vi "运维调试_CODMn.vi"() -> ()   [LabVIEW 2016, in "斯坦道CODMn新电路板.lvlib"]
uses:
  <vilib>/Utility/miscctls.llb/LVPointTypeDef.ctl
  <vilib>/Waveform/WDTFileIO.llb/Read Waveform from File.vi
  <vilib>/ptbypt/NI_PtbyPt.lvlib
panel:
  in  "告警代码":u16
  in  "周期设置":bool
  out "消解压力kPa":sgl format="%#.2f"
  out "权限等级":string
  out "总步数":i32
  out "滑动杆":u8(slide) caption="测试进度" scale=0.0..100.0
  in  "参数查询":bool
  in  "仪器校准":bool
  out "仪器版本号":string
  in  "试剂余量设置":bool
  out "试剂余量显示":sgl[][](graph)
  in  "公式切换阈值滴定数(0~9999)":dbl
  out "X0":u16
  in  "平台反控标样校准":enum16{"标液1", "标液2", "标液3"}(ring)
  in  "平台反控校准量程":enum16{"低量程1", "低量程2", "高量程1", "高量程2"}(ring)
  out "试剂传感器":sgl format="%#.2f"
  in  "历史波形 2":bool
  in  "返回 3":bool
  out "时间-温度":u16[](array[numeric]) caption="数组"
  out "温度波形时间":timestamp
  out "ORP滴定曲线 2":u16[](graph)
  in  "历史波形":bool
  in  "返回 2":bool
  out "滴定数-ORP值":u16[](array[numeric]) caption="数组"
  out "波形时间":timestamp
  out "ORP滴定曲线":u16[](graph)
  in  "滴定曲线":bool
  out "终点滴定数":sgl format="%#.2f"
  out "单位:":T1(ring)
  out "运行状态":T2 {"数据时间:" format="%<%y/%m/%d %H:%M:%S>T"; "仪器时间:" format="%<%y/%m/%d %H:%M:%S>T"}
  out "模块版本号":string
  out "当前步骤剩余时间":sgl format="%#.2f"
  out "加热实时温度":sgl format="%#.2f"
  out "ORP值/光值":sgl format="%#.2f"
  in  "布尔":bool
  in  "流程固件":bool
  in  "公式单个写入":bool
  in  "流程路径":path=path "C:/Users/STD/Documents/斯坦道流程文件/流程.xml"
  out "字符串":string
  out "运行时间":sgl format="%#.2f"
  out "环境湿度":sgl format="%#.2g"
  out "环境温度":sgl format="%#.2g"
  in  "数组":string[](array[string])
  in  "量程切换阈值写入":bool
  in  "量程切换阈值读取":bool
  in  "参数下拉列表":enum16{"CODMn"}(ring)
  in  "量程下拉列表":enum16{"低量程1", "低量程2", "高量程1", "高量程2"}(ring)
  in  "测量模式下拉列表":T3(ring)=enum."水样测量"
  in  "公式":cluster{"X^2":dbl, "X":dbl, "b":dbl}
  in  "写公式":bool
  in  "读公式":bool
  in  "返回":bool
  in  "设置":bool
  out "集成报警信息":string
  in  "停止":bool
  in  "手动启动":bool
  in  "单步测试":bool
  out "当前滴定数":sgl format="%#.2f"
  out "K":sgl format="%#.2f"
  out "B":sgl format="%#.2f"
  out "A":sgl format="%#.2f"
  out "多列列表框":i32(listbox)
  # "."
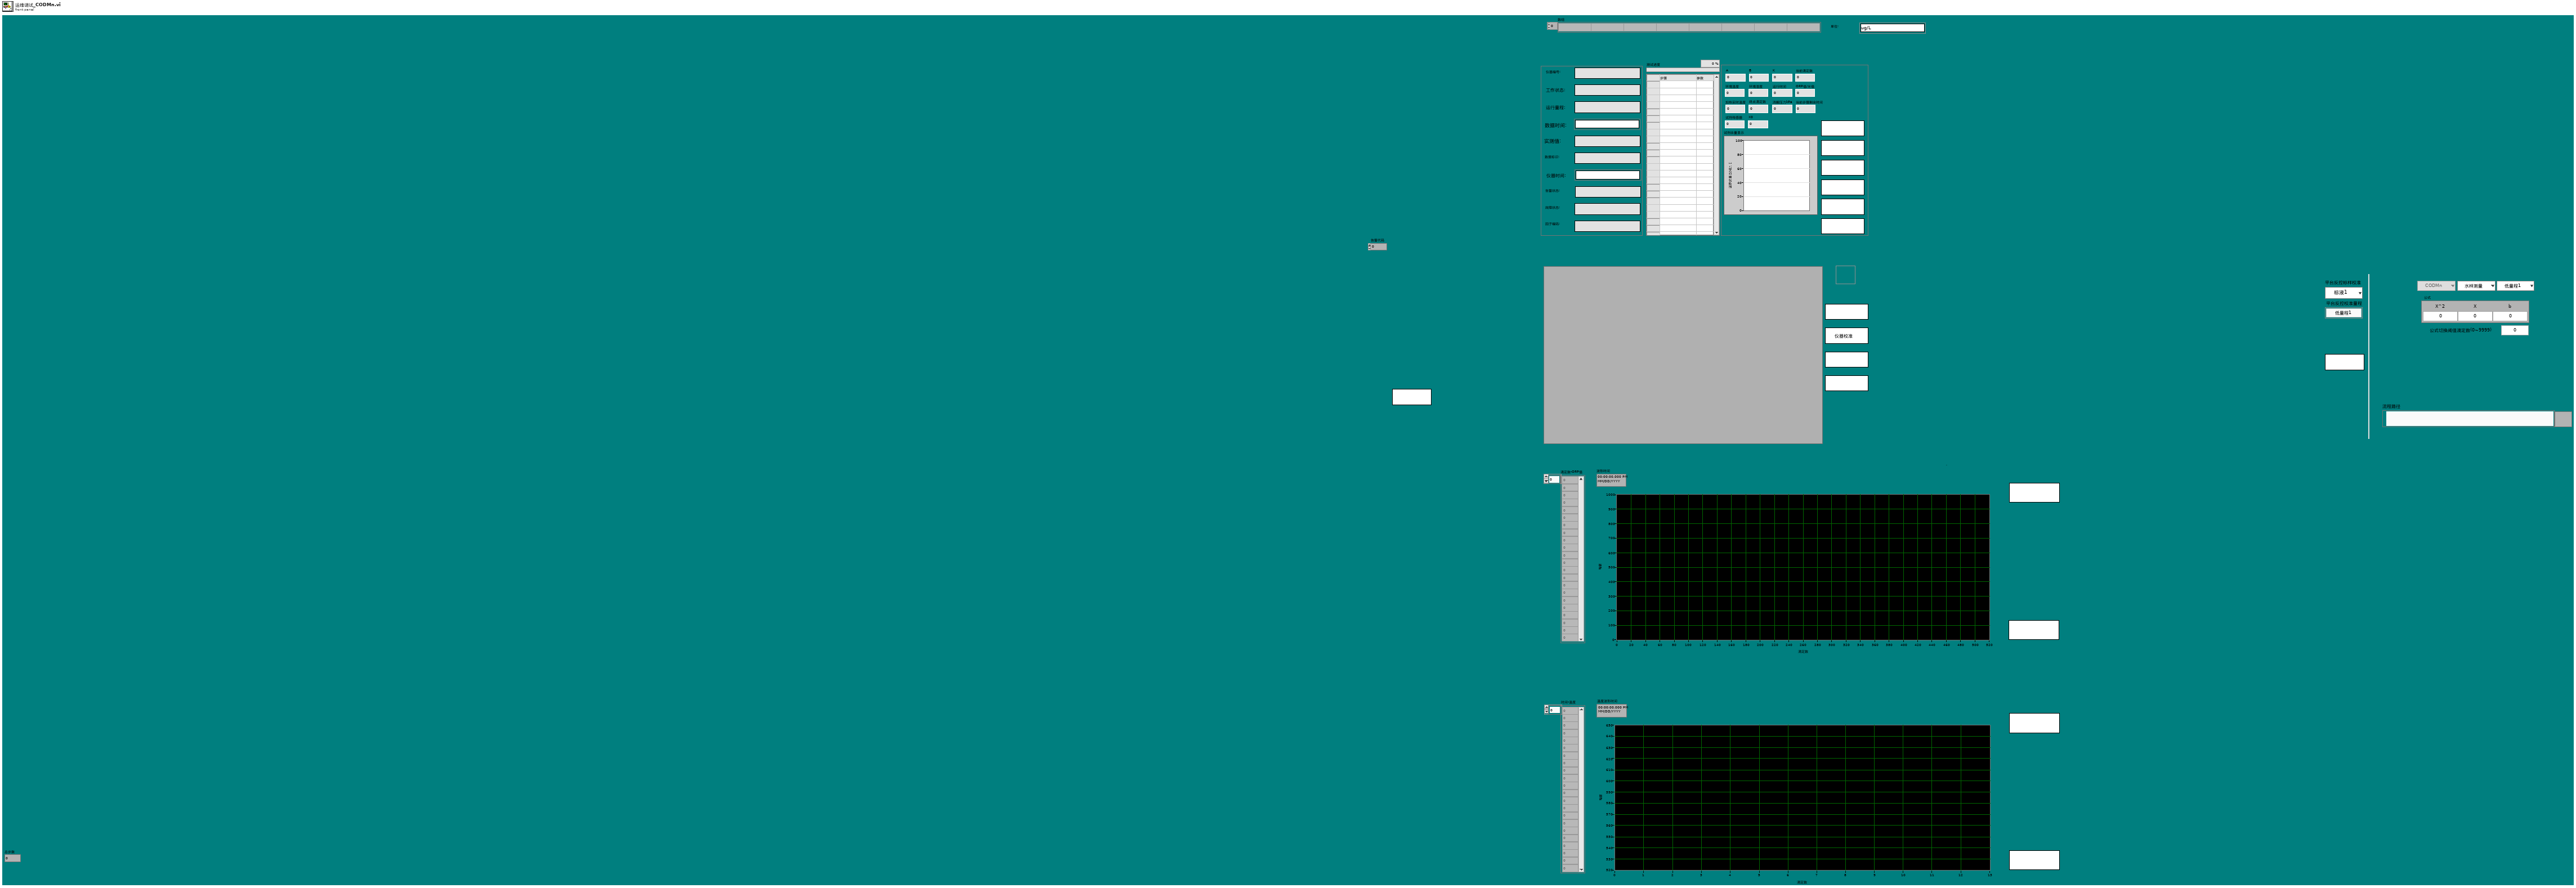
[diagram p1: front panel]
types:
  T1 = enum16{"ug/L", "mg/L", "ppm", "mg/m3", "cm", "ppb", "ug/m3", "%", "nmol/mol", "umol/mol", "MPN/L", "MPN/100ml", "ng/m3", "NTU", "无量纲", "ms/cm", "us/cm", "℃", "mV", "万个/L"}
  T2 = cluster{"仪器编号:":string, "工作状态:":string, "运行量程: ":string, "数据时间:":timestamp, "实测值:":string, "数据标识: ":string, "仪器时间:":timestamp, "告警状态: ":string, "故障状态:  ":string, "因子编码:":string}
  T3 = enum16{"", "水样测量", "标样核查", "零点核查", "跨度核查", "空白测试", "平行样测试", "加标回收"}
  T4 = cluster{"Major":u16, "Minor":u16, "Fix":u16, "Build":u16}
  T5 = cluster{"测量量程":sgl, "测量检出限":sgl, "测量精度":sgl, "测量间隔":sgl, "消解温度":sgl, "消解时长":sgl, "三项式系数":sgl, "二次多项式系数":sgl, "曲线斜率":sgl, "曲线截距":sgl, "线性相关系数":sgl, "空白校准时间":timestamp, "标样校准时间":timestamp, "测量信号值":sgl, "稀释倍数":sgl, "量程系数":sgl}
  T6 = typedef "LVPointTypeDef.ctl" = cluster{"Horizontal":i16, "Vertical":i16}
  T7 = cluster{"因子编码":u32, "单位":u16, "标样参考值":sgl, "水样数据时间":timestamp, "水样实测值":sgl, "水样数据标识":string, "标样数据时间":timestamp, "标样实测值":sgl, "标样数据标识":string, "空白数据时间":timestamp, "空白实测值":sgl, "空白数据标识":string, "零点核查数据时间":timestamp, "零点核查实测值":sgl, "零点核查数据标识":string, "跨度核查数据时间":timestamp, "跨度核查实测值":sgl, "跨度核查数据标识":string, "加标回收数据时间":timestamp, "加标回收实测值":sgl, "加标回收数据标识":string, "平行样数据时间":timestamp, "平行样实测值":sgl, "平行样数据标识":string, "F0":sgl, "F1":sgl, "F2":sgl, "F3":sgl, "F4":sgl, "F5":sgl, "F6":sgl, "F7":sgl, "温度":sgl, "湿度":sgl, "X值":sgl, "fidrange":u16}
  T8 = cluster{"系统时间":timestamp, "工作状态":u16, "测量模式":enum16{"待机", "连续模式", "周期模式", "定点模式", "受控模式", "手动模式"}, "告警代码":u16, "故障代码":u16, "日志代码":u16, "软件版本":u16, "A":sgl, "B":sgl, "K":sgl, "当前滴定数":sgl, "T":sgl, "H":sgl, "id":u16, "flowid":u16, "量程":u16, "加热实时温度":sgl, "当前ORP值":sgl, "运行时间":sgl, "当前步骤剩余时间":sgl, "结束滴定数":sgl, "注射泵保温温度":sgl, "匹配滴定数X0":u16, "X^2":sgl, "X":sgl, "B 2":sgl, "光值1":sgl, "光值2":sgl, "光值3":sgl, "光值4":sgl, "光值5":sgl, "光值6":sgl, "光值7":sgl, "光值8":sgl}
  T9 = cluster{"id":string, "ver":string, "type":string, "code":u16, "level":enum16{"一级", "二级", "三级"}, "message":string, "analysis":string, "platform_alarm_code":string}
  T10 = enum8{"Enabled", "Disabled", "Disabled and Grayed Out"}
  T11 = enum16{"空闲", "水样测试", "标样核查", "零点核查", "跨度核查", "空白测试", "平行样测试", "加标回收", "空白校准", "标样校准", "初始化（清洗）"}
  T12 = typedef "TimingControl.lvlib/TimingControl.lvclass/国标控制命令.ctl" = enum16{"启动测量", "标样核查", "零点核查", "跨度核查", "空白测试", "平行样测试", "加标回收", "空白校准", "标样校准", "初始化（清洗）", "停止测试", "仪器重启", "校时", "模式设置", "测量间隔设置"}
  T13 = typedef "TimingControl.lvlib/TimingControl.lvclass/测量参数.ctl" = u16
  T14 = cluster{"时间标识":timestamp, "设备":string, "日志信息":string, "流程参数":string}
  T15 = typedef "LVRowAndColumnUnsignedTypeDef.ctl" = cluster{"Row":u32, "Column":u32}
  T16 = enum32{"Bad", "Idle", "Run top level", "Running"}
  T17 = cluster{"站号":u16, "量程切换":enum32{"H", "L", "AUTO"}, "控制命令":u16, "模式设置":enum16{"待机", "连续模式", "周期模式", "定点模式", "受控模式", "手动模式"}, "测量间隔":u16}
  T18 = cluster{"测量量程":dbl, "测量精度":dbl, "测量间隔":dbl, "消解温度":dbl, "消解时长":dbl, "空白校准时间":timestamp, "曲线截距":dbl, "曲线斜率":dbl, "测量检出限":dbl, "测量信号值":dbl, "线性相关系数":dbl, "二次多项式系数":dbl, "标样校准时间":timestamp, "稀释倍数":dbl, "三项式系数":dbl, "空白标定系数":dbl, "量程系数":dbl, "F0/ORPA":dbl, "F1/ORPB":dbl, "F2/ORPK":dbl, "F3":dbl, "F4":dbl, "F5":dbl, "F6":dbl, "F7":dbl, "X0/滴定数":dbl, "量程":dbl}
  T19 = cluster{"跨度值":dbl, "零点标准液浓度":dbl, "跨度标准液浓度":dbl, "标准液标准浓度":dbl, "零点标准液偏差":dbl, "跨度标准液偏差":dbl, "标准液标准偏差":dbl}
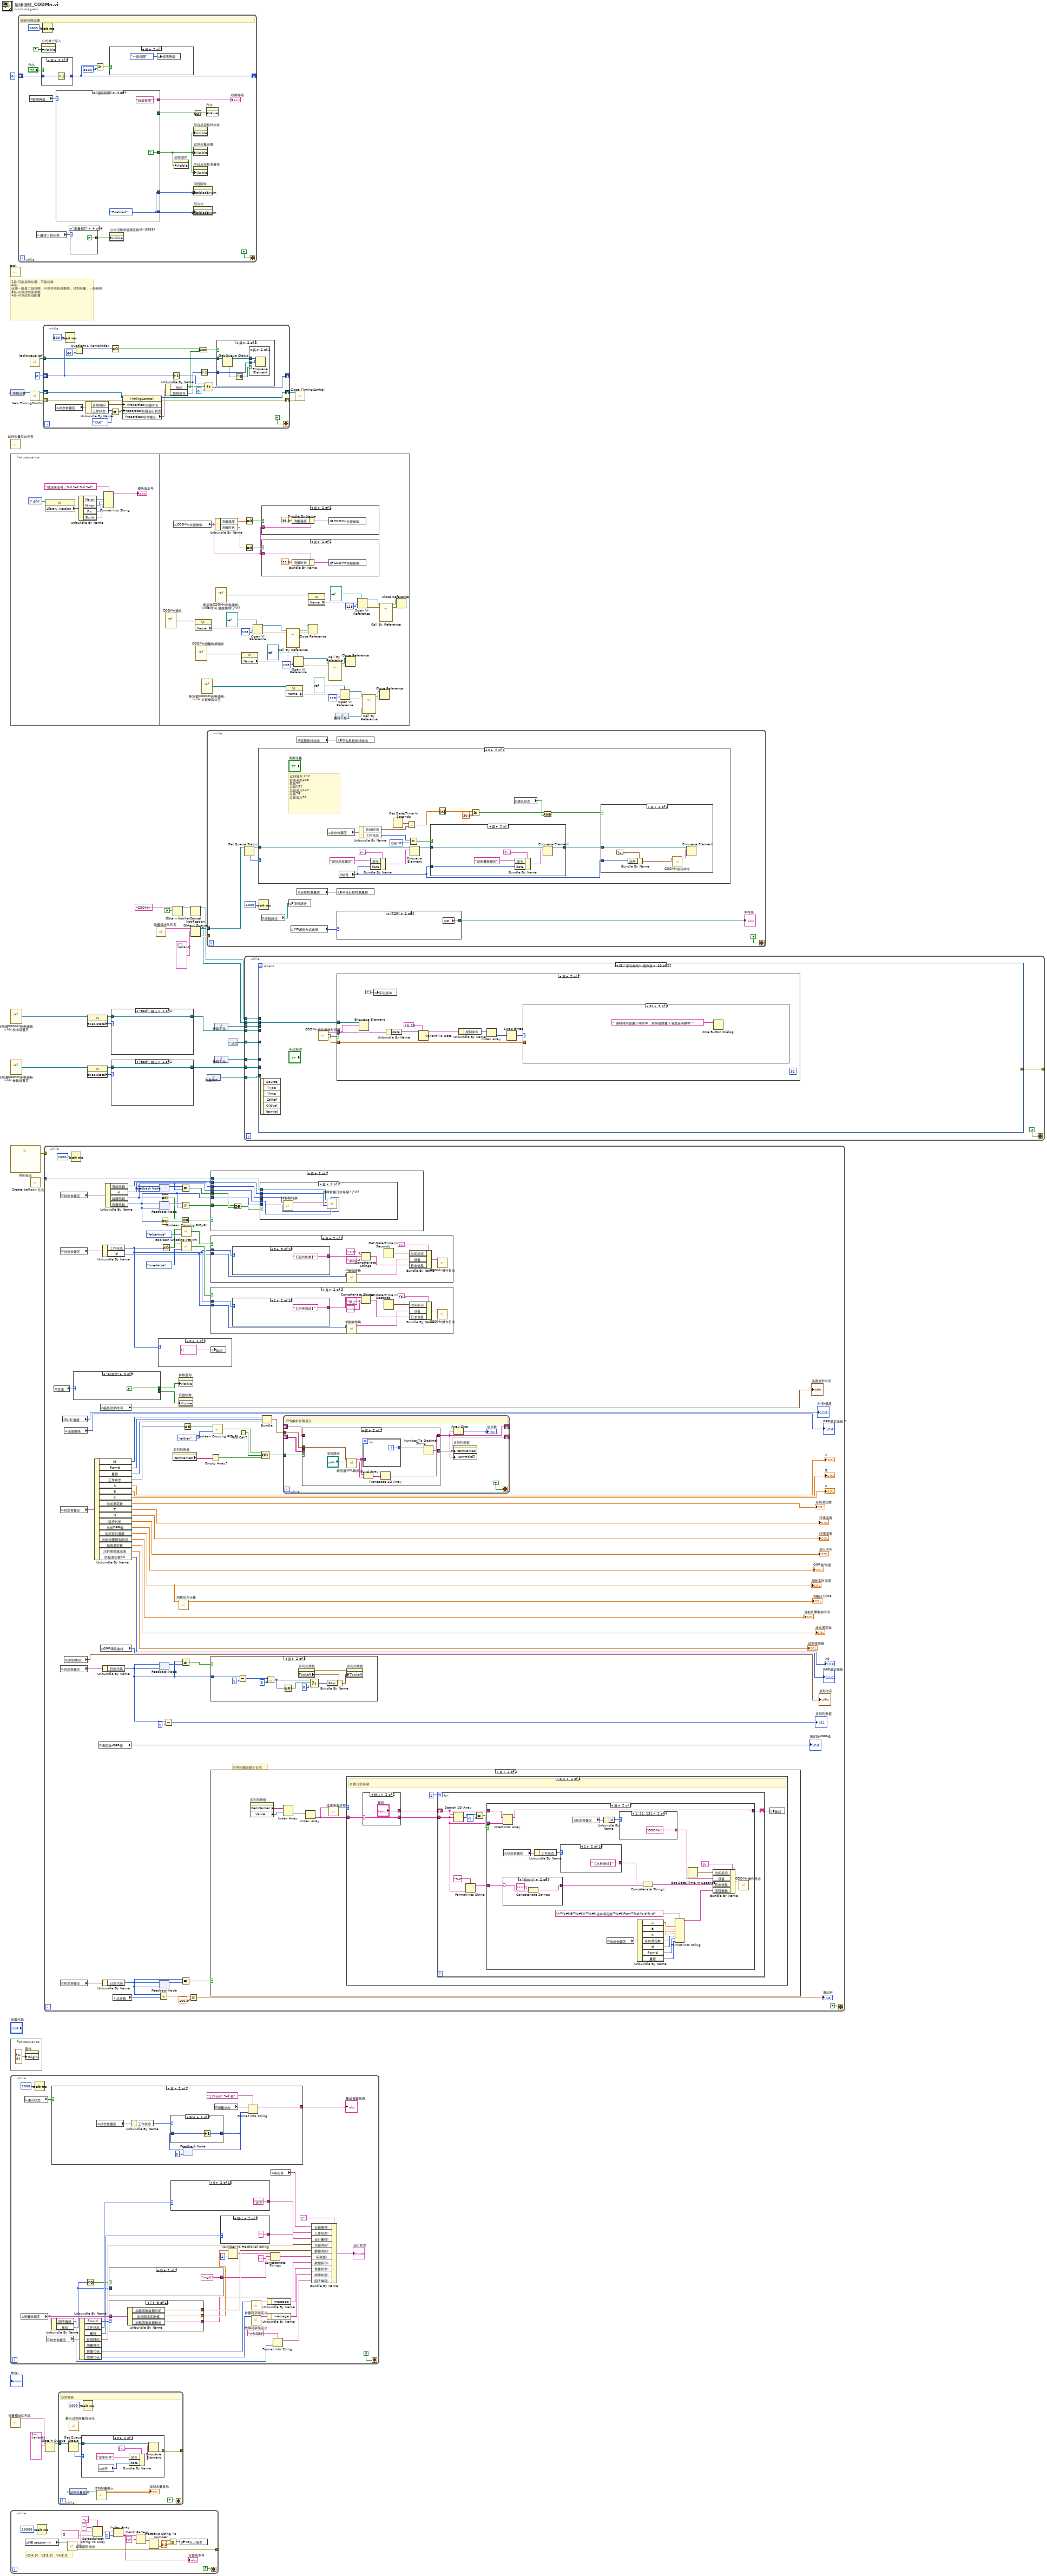
[diagram p0: block diagram]
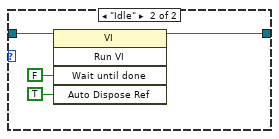
[diagram p2: hidden frame]
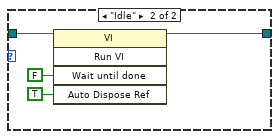
[diagram p3: hidden frame]
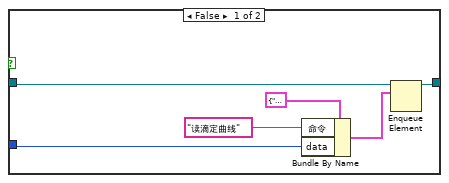
[diagram p6: hidden frame]
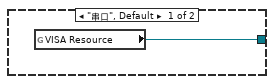
[diagram p8: hidden frame]
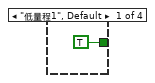
[diagram p11: hidden frame]
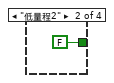
[diagram p12: hidden frame]
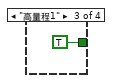
[diagram p13: hidden frame]
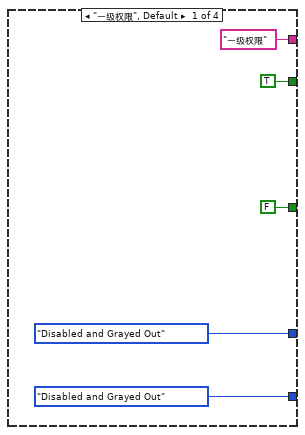
[diagram p14: hidden frame]
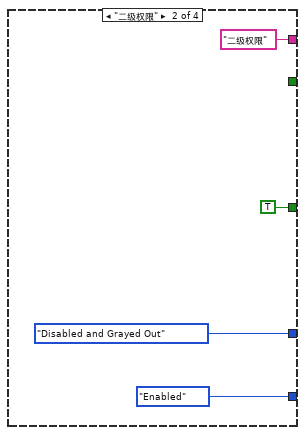
[diagram p15: hidden frame]
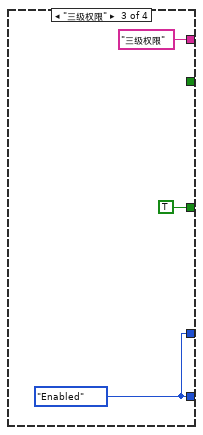
[diagram p16: hidden frame]
diagram:
  # "1级.只能启动仪器，不能校准\n2级.运维一般是二级权限，可以校准和改曲线，试剂余量，一般参数\n3级.可以改内部参数\n4级.可以改外设配置"
  n1 = call "task.vi"() -> ()  [unwired: 12 in]
  n2 = control-ref of="周期设置"() -> (w5:refnum<vi>)
  n3 = call "试剂余量后台任务.vi"() -> ()  [unwired: 12 in]
  n4 = flat-sequence {
    frame #0 {
      n5 = control-ref of="本VI"() -> (w41:refnum<vi>)
      n6 = property class="VI"(reference=w41) -> ("Library.Version"=w40:T4)  [unwired: 1 in, 2 out]
      n7 = Unbundle By Name(w40) -> ("Major"=w38:u16, "Minor"=w37:u16, "Fix"=w36:u16, "Build"=w35:u16)
      n8 = Format Into String(format string="模块版本号：%d.%d.%d.%d" ("格式字符串"), w38, w37, w36, w35) -> (resulting string=→"模块版本号":string)  [unwired: 2 in, 1 out]
    }
    frame #1 {
      n9 = vi-ref "CODMn通讯.vi"() -> (w55:refnum<vi>)
      n10 = global read "CODMn断电保存全局变量.vi" "CODMn关键参数"() -> (w42:T5)
      n11 = property class="VI"(reference=w55) -> ("Name"=w54:string)  [unwired: 1 in, 2 out]
      n12 = vi-ref "CODMn测量数据储存.vi"() -> (w79:refnum<vi>)
      n13 = vi-ref "斯坦道CODMn新电路板.lvlib:关键参数交互.vi"() -> (w65:refnum<vi>)
      n14 = Unbundle By Name(w42) -> ("消解温度"=w46:sgl, "消解时长"=w43:sgl)
      n15 = vi-ref "斯坦道CODMn新电路板.lvlib:时间-温度曲线(子VI).vi"() -> (w57:refnum<vi>)
      n16 = property class="VI"(reference=w79) -> ("Name"=w72:string)  [unwired: 1 in, 2 out]
      n17 = Equal To 0?(x=w46) -> (x = 0?=w45:bool)
      n18 = Equal To 0?(x=w43) -> (x = 0?=w44:bool)
      n19 = Open VI Reference(type specifier VI Refnum (for type only)=refnum<vi> refnum, vi path=w54, options=128 ("选项")) -> (vi reference=w52:refnum<vi>, error out=w50:errorcluster)  [unwired: 3 in]
      n20 = case shown="真" w45 {
        tunnel: w42 -> [_ w85]
        frame False {
        }
        frame True {
          n21 = Bundle By Name(cluster=w85, "消解温度"=sgl 95.0) -> (w84:T5)
          n22 = global write "CODMn断电保存全局变量.vi" "CODMn关键参数"(w84) -> ()
        }
      }
      n23 = case shown="真" w44 {
        tunnel: w42 -> [_ w82]
        frame False {
        }
        frame True {
          n24 = Bundle By Name(cluster=w82, "消解时长"=sgl 25.0) -> (w81:T5)
          n25 = global write "CODMn断电保存全局变量.vi" "CODMn关键参数"(w81) -> ()
        }
      }
      n26 = property class="VI"(reference=w65) -> ("Name"=w71:string)  [unwired: 1 in, 2 out]
      n27 = call-by-ref "?"(reference=w52, error in=w50) -> (reference out=w48:refnum<vi>, error out=w49:errorcluster)  [unwired: 12 in]
      n28 = Open VI Reference(type specifier VI Refnum (for type only)=refnum<vi> refnum, vi path=w72, options=128 ("选项")) -> (vi reference=w74:refnum<vi>, error out=w76:errorcluster)  [unwired: 3 in]
      n29 = property class="VI"(reference=w57) -> ("Name"=w63:string)  [unwired: 1 in, 2 out]
      n30 = Close Reference(reference=w48, error in (no error)=w49) -> ()  [unwired: 1 out]
      n31 = call-by-ref "?"(reference=w74, error in=w76) -> (reference out=w78:refnum<vi>, error out=w77:errorcluster)  [unwired: 12 in]
      n32 = control-ref of="量程下拉列表"() -> (w47:refnum<vi>)
      n33 = Open VI Reference(type specifier VI Refnum (for type only)=refnum<vi> refnum, vi path=w71, options=128 ("选项")) -> (vi reference=w69:refnum<vi>, error out=w68:errorcluster)  [unwired: 3 in]
      n34 = Close Reference(reference=w78, error in (no error)=w77) -> ()  [unwired: 1 out]
      n35 = Open VI Reference(type specifier VI Refnum (for type only)=refnum<vi> refnum, vi path=w63, options=128 ("选项")) -> (vi reference=w61:refnum<vi>, error out=w60:errorcluster)  [unwired: 3 in]
      n36 = call-by-ref "?"(reference=w69, error in=w68, "量程下拉列表"=w47) -> (reference out=w66:refnum<vi>, error out=w67:errorcluster)  [unwired: 11 in]
      n37 = call-by-ref "?"(reference=w61, error in=w60) -> (reference out=w58:refnum<vi>, error out=w59:errorcluster)  [unwired: 12 in]
      n38 = Close Reference(reference=w66, error in (no error)=w67) -> ()  [unwired: 1 out]
      n39 = Close Reference(reference=w58, error in (no error)=w59) -> ()  [unwired: 1 out]
    }
  }
  n40 = vi-ref "斯坦道CODMn新电路板.lvlib:校准设置页.vi"() -> (w17:refnum<vi>)
  n41 = vi-ref "斯坦道CODMn新电路板.lvlib:参数设置页.vi"() -> (w14:refnum<vi>)
  n42 = call "时间延迟"() -> ("error out"=w27:errorcluster)  [unwired: 11 in]
  n43 = flat-sequence {
    frame #0 {
      n44 = property on="窗格" class="Pane"("Origin"=T6 {"Horizontal"=0, "Vertical"=0} ("原点")) -> ()  [unwired: 2 in, 2 out]
    }
  }
  n45 = while {
    stop <- FALSE stop-if-true
    n46 = global read "VARCODMn全局变量.vi" "测量数据区"() -> (w114:T7)
    n47 = global read "VARCODMn全局变量.vi" "通讯状态"() -> (w118:bool)
    n48 = Wait (ms)(milliseconds to wait=u32 1000 ("等待时间（毫秒）")) -> ()  [unwired: 1 out]
    n49 = global read "VARCODMn全局变量.vi" "状态告警区"() -> (w116:T8)
    n50 = case shown="真" w118 {
      tunnel: ["通讯异常" ("集成报警信息") w196] -> w117
      frame False {
      }
      frame True {
        n51 = global read "VARCODMn全局变量.vi" "状态告警区"() -> (w202:T8)
        n52 = Unbundle By Name(w202) -> ("工作状态"=w201:u16)
        n53 = feedback #1(0) -> (w199:i32)
        n54 = case shown="默认" w201 {
          tunnel: w199 -> [_ w204]
          tunnel: [_ w203] -> w197
          frame 0 {
          }
          frame Default {
            n55 = Increment(x=w204) -> (x+1=w203:i32)
          }
        }
        n56 = feedback-in #1(w197) -> ()
        n57 = global read "VARCODMn全局变量.vi" "测量状态"() -> (w195:string)
        n58 = Format Into String(format string="工作计时: %d 秒" ("格式字符串"), initial string=w195, w197) -> (resulting string=w196:string)  [unwired: 1 in, 1 out]
      }
    }
    "集成报警信息" <- w117
    n59 = Unbundle By Name(w114) -> ("因子编码"=w94:u32, "单位"=w91:u16)
    n60 = Unbundle By Name(w116) -> ("flowid"=w115:u16, "工作状态"=w112:u16, "量程"=w110:u16, "系统时间"=w108:timestamp, "告警代码"=w98:u16, "故障代码"=w97:u16)  [unwired: 1 out]
    n61 = Not Equal To 0?(x=w91) -> (x != 0?=w92:bool)
    n62 = case shown="假" w92 {
      tunnel: ["mg/L" ("RingText.Text") w123] -> w96
      tunnel: w91 -> [_ w122]
      frame False {
      }
      frame True {
        n63 = property on="单位:" class="Enum (严格)"("Value"=w122) -> (error out=w124:errorcluster)  [unwired: 2 in, 1 out]
        n64 = property on="单位:" class="Enum (严格)"(error in=w124) -> ("RingText.Text"=w123:string)  [unwired: 1 in, 2 out]
      }
    }
    n65 = case shown="7" w115 {
      selector: w115 -> [w147 _ _ _ _ _ _ _ _ _ _ _]
      tunnel: [_ w153 w157 w161 w165 w169 w173 w177 w181 w184 w188 w193] -> w105
      tunnel: [_ w151 w156 w160 w164 w168 w172 w175 w180 w183 w187 w192] -> w100
      tunnel: [_ w150 w155 w159 w163 w167 w171 w174 w179 w182 w186 w191] -> w99
      tunnel: w114 -> [_ w152 w154 w158 w162 w166 w170 w176 w178 w185 w189 w190]
      frame Default {
        n66 = Format Into String(format string="%d" ("格式字符串"), initial string="未知" ("工作状态"), w147) -> ()  [unwired: 1 in, 2 out]
      }
      frame 0 {
        n67 = Unbundle By Name(w152) -> ("水样数据时间"=w153:timestamp, "水样实测值"=w151:sgl, "水样数据标识"=w150:string)
      }
      frame 1 {
        n68 = Unbundle By Name(w154) -> ("水样数据时间"=w157:timestamp, "水样实测值"=w156:sgl, "水样数据标识"=w155:string)
      }
      frame 2 {
        n69 = Unbundle By Name(w158) -> ("标样数据时间"=w161:timestamp, "标样实测值"=w160:sgl, "标样数据标识"=w159:string)
      }
      frame 3 {
        n70 = Unbundle By Name(w162) -> ("零点核查数据时间"=w165:timestamp, "零点核查实测值"=w164:sgl, "零点核查数据标识"=w163:string)
      }
      frame 4 {
        n71 = Unbundle By Name(w166) -> ("跨度核查数据时间"=w169:timestamp, "跨度核查实测值"=w168:sgl, "跨度核查数据标识"=w167:string)
      }
      frame 5 {
        n72 = Unbundle By Name(w170) -> ("空白数据时间"=w173:timestamp, "空白实测值"=w172:sgl, "空白数据标识"=w171:string)
      }
      frame 6 {
        n73 = Unbundle By Name(w176) -> ("平行样数据时间"=w177:timestamp, "平行样实测值"=w175:sgl, "平行样数据标识"=w174:string)
      }
      frame 7 {
        n74 = Unbundle By Name(w178) -> ("加标回收数据时间"=w181:timestamp, "加标回收实测值"=w180:sgl, "加标回收数据标识"=w179:string)
      }
      frame 8 {
        n75 = Unbundle By Name(w185) -> ("空白数据时间"=w184:timestamp, "空白实测值"=w183:sgl, "空白数据标识"=w182:string)
      }
      frame 9 {
        n76 = Unbundle By Name(w189) -> ("标样数据时间"=w188:timestamp, "标样实测值"=w187:sgl, "标样数据标识"=w186:string)
      }
      frame 10 {
        n77 = Unbundle By Name(w190) -> ("水样数据时间"=w193:timestamp, "水样实测值"=w192:sgl, "水样数据标识"=w191:string)
      }
    }
    n78 = case shown="0" w112 {
      selector: w112 -> [w128 _ _ _ _ _ _ _ _ _ _ _ _ _ _ _]
      tunnel: [w129 "空闲" ("工作状态") "水样测量" ("工作状态") "标样核查" ("工作状态") "零点核查" ("工作状态") "跨度核查" ("工作状态") "空白测试" ("工作状态") "平行样测试" ("工作状态") "加标回收" ("工作状态") "空白校准" ("工作状态") "标样校准" ("工作状态") "初始化" ("工作状态") "调试" ("工作状态") "填充管路" ("工作状态") "清洗管路" ("工作状态") "清洗反应杯" ("工作状态")] -> w111
      frame Default {
        n79 = Format Into String(format string="%d" ("格式字符串"), initial string="未知" ("工作状态"), w128) -> (resulting string=w129:string)  [unwired: 1 in, 1 out]
      }
      frame 0 {
      }
      frame 1 {
      }
      frame 2 {
      }
      frame 3 {
      }
      frame 4 {
      }
      frame 5 {
      }
      frame 6 {
      }
      frame 7 {
      }
      frame 8 {
      }
      frame 9 {
      }
      frame 10 {
      }
      frame 22 {
      }
      frame 30 {
      }
      frame 31 {
      }
      frame 32 {
      }
    }
    n80 = case shown="默认" w110 {
      tunnel: ["" ("字符串") "低量程" ("字符串") "高量程" ("字符串")] -> w109
      frame Default {
      }
      frame 0 {
      }
      frame 1 {
      }
    }
    n81 = Number To Fractional String(number=w100, precision (6)=i16 2 ("精度(6)")) -> (F-format string=w103:string)  [unwired: 2 in]
    n82 = call "告警码字段定义.vi"("告警代码"=w98) -> ("报警信息"=w90:T9)  [unwired: 10 in]
    n83 = call "故障码字段定义.vi"("故障代码"=w97) -> ("故障信息"=w89:T9)  [unwired: 10 in]
    n84 = Unbundle By Name(w90) -> ("message"=w87:string)
    n85 = Unbundle By Name(w89) -> ("message"=w88:string)
    n86 = Concatenate Strings(w103, " " ("字符串"), w96) -> (w101:string)
    n87 = global read "VARCODMn全局变量.vi" "序列号"() -> (w113:string)
    n88 = Format Into String(format string="w%05d" ("格式字符串"), w94) -> (resulting string=w93:string)  [unwired: 2 in, 1 out]
    n89 = Bundle By Name(cluster=T2 {"仪器编号:"="", "工作状态:"="", "运行量程: "="", "数据时间:"=timestamp(0 s since 1904-01-01), "实测值:"="", "数据标识: "="", "仪器时间:"=timestamp(0 s since 1904-01-01), "告警状态: "="", "故障状态:  "="", "因子编码:"=""} ("运行状态"), "仪器编号:"=w113, "工作状态:"=w111, "运行量程:"=w109, "仪器时间:"=w108, "数据时间:"=w105, "实测值:"=w101, "数据标识:"=w99, "告警状态:"=w87, "故障状态:"=w88, "因子编码:"=w93) -> (→"运行状态":T2)
  }
  n90 = call "设置模块队列名.vi"() -> ("Msg"=w6:string)  [unwired: 11 in]
  n91 = while {
    tunnel: [w217] -> _
    stop <- FALSE stop-if-true
    # "V2(4.0)   V3(5.0)   V4(6.0)"
    n92 = global read "VARCODMn全局变量.vi" "MB session in"() -> (w218:refnum<class "MB_Master.lvclass">)
    n93 = Wait (ms)(milliseconds to wait=u32 10000 ("等待时间（毫秒）")) -> ()  [unwired: 1 out]
    n94 = call "读取固件状态.vi"("MB session in"=w218) -> ("error out"=w217:errorcluster, "结果字符串"=w213:string)  [unwired: 8 in, 1 out]
    n95 = Spreadsheet String To Array(delimiter (Tab)="\n" ("分隔符(Tab)"), format string="" ("格式字符串"), spreadsheet string=w213, array type (2D Dbl)=string[] []) -> (array=w212:string[])
    n96 = Index Array(array=w212, index=1 ("索引")) -> (element=w205:string)
    "仪器版本号" <- w205
    n97 = Match Pattern(string=w205, regular expression="V" ("正则表达式")) -> (after substring=w209:string)  [unwired: 1 in, 3 out]
    n98 = Fract/Exp String To Number(string=w209) -> (number=w208:dbl)  [unwired: 3 in, 1 out]
    n99 = Greater Or Equal?(x=w208, y=5.0) -> (x >= y?=w206:bool)
    n100 = global write "VARCODMn全局变量.vi" "V5以上版本"(w206) -> ()
  }
  n101 = while {
    shift-right: [w234] -> _
    shift-left: u32 0 ("等待时间（毫秒）") -> [w235]
    stop <- FALSE stop-if-true
    # "密码权限设置"
    n102 = global read "VARCODMn全局变量.vi" "权限等级"() -> (w226:enum16{"一级权限", "二级权限", "三级权限", "超级权限"})
    n103 = local read "量程下拉列表"() -> (w228:enum16{"低量程1", "低量程2", "高量程1", "高量程2"})
    n104 = property on="公式单个写入" class="Bool"("Visible"=FALSE ("可见")) -> ()  [unwired: 2 in, 2 out]
    n105 = case shown="真" "布尔" {
      tunnel: w235 -> [_ w259]
      tunnel: [_ w258] -> w234
      frame False {
      }
      frame True {
        n106 = Increment(x=w259) -> (x+1=w258:u32)
      }
    }
    n107 = Wait (ms)(milliseconds to wait=u32 1000 ("等待时间（毫秒）")) -> ()  [unwired: 1 out]
    n108 = case shown="\"超级权限\"" w226 {
      tunnel: [T10."Disabled and Grayed Out" ("f") T10."Enabled" ("禁用") w253 w256] -> w229
      tunnel: [T10."Disabled and Grayed Out" ("f") T10."Disabled and Grayed Out" ("f") w253 w256] -> w230
      tunnel: [FALSE ("可见") TRUE ("可见") TRUE ("可见") TRUE ("可见")] -> w225
      tunnel: ["一级权限" "二级权限" "三级权限" "超级权限"] -> w224
      tunnel: [TRUE _ _ _] -> w223
      frame "一级权限", Default {
      }
      frame "二级权限" {
      }
      frame "三级权限" {
        w253 = T10."Enabled" ("禁用")
      }
      frame "超级权限" {
        w256 = T10."Enabled" ("禁用")
      }
    }
    "权限等级" <- w224
    n109 = case shown="\"高量程2\"" w228 {
      tunnel: [TRUE ("可见") FALSE ("可见") TRUE ("可见") FALSE ("可见")] -> w227
      frame "低量程1", Default {
      }
      frame "低量程2" {
      }
      frame "高量程1" {
      }
      frame "高量程2" {
      }
    }
    n110 = Greater Or Equal?(x=w234, y=u32 3600) -> (x >= y?=w232:bool)
    n111 = case shown="真" w232 {
      frame False {
      }
      frame True {
        n112 = global write "VARCODMn全局变量.vi" "权限等级"(enum16{"一级权限", "二级权限", "三级权限", "超级权限"}."一级权限" ("权限等级")) -> ()
      }
    }
    n113 = property on="公式切换阈值滴定数(0~9999)" class="DigNum (严格)"("Visible"=w227) -> ()  [unwired: 2 in, 2 out]
    n114 = property on="流程固件" class="Bool"("Visible"=w225) -> ()  [unwired: 2 in, 2 out]
    n115 = Not(x=w223) -> (.not. x?=w221:bool)
    n116 = property on="平台反控标样校准" class="Enum (严格)"("Visible"=w225) -> ()  [unwired: 2 in, 2 out]
    n117 = property on="试剂余量设置" class="Bool"("Visible"=w225) -> ()  [unwired: 2 in, 2 out]
    n118 = property on="平台反控校准量程" class="Enum (严格)"("Visible"=w225) -> ()  [unwired: 2 in, 2 out]
    n119 = property on="流程固件" class="Bool"("DisabledEnum"=w230) -> ()  [unwired: 2 in, 2 out]
    n120 = property on="写公式" class="Bool"("DisabledEnum"=w229) -> ()  [unwired: 2 in, 2 out]
    n121 = property on="布尔" class="Bool (严格)"("Value"=w221) -> ()  [unwired: 2 in, 2 out]
  }
  n122 = call "taskqueue ref.vi"() -> ("队列输出"=w9:refnum<queue>)  [unwired: 10 in, 1 out]
  n123 = call "New TimingControl.vi"("Reference"=w5) -> ("error out"=w3:errorcluster, "TimingControl out"=w4:refnum<class "TimingControl.lvclass">)  [unwired: 9 in]
  n124 = call "Create balloon 队列.vi"() -> ("队列输出"=w20:refnum<queue>)  [unwired: 11 in]
  n125 = while {
    tunnel: w9 -> [w279]
    shift-right: [w269] -> _
    shift-left: u32 0 ("等待时间（毫秒）") -> [w270]
    shift-right: [w264] -> w2
    shift-left: w4 -> [w266]
    shift-right: [w263] -> w1
    shift-left: w3 -> [w265]
    stop <- FALSE stop-if-true
    n126 = global read "VARCODMn全局变量.vi" "状态告警区"() -> (w281:T8)
    n127 = Wait (ms)(milliseconds to wait=u32 500 ("等待时间（毫秒）")) -> ()  [unwired: 1 out]
    n128 = Quotient & Remainder(x=w270, y=u32 60) -> (x-y*floor(x/y)=w267:u32)  [unwired: 1 out]
    n129 = Unbundle By Name(w281) -> ("系统时间"=w261:timestamp, "工作状态"=w274:u16)
    n130 = Equal To 0?(x=w267) -> (x = 0?=w276:bool)
    n131 = Not Equal?(x=w274, y=T11."空闲") -> (x != y?=w260:bool)
    n132 = property class="TimingControl"(reference=w266, error in=w265, "Properties:仪器时间"=w261, "Properties:仪器运行状态"=w260) -> (reference out=w264:refnum<class "TimingControl.lvclass">, error out=w263:errorcluster, "Properties:命令输出"=w262:cluster{"启动":bool, "控制命令":T12, "测量参数":T13})
    n133 = Unbundle By Name(w262) -> ("启动"=w273:bool, "控制命令"=w278:T12)
    n134 = Increment(x=w270) -> (x+1=w272:u32)
    n135 = And(x=w276, y=w273) -> (x .and. y?=w275:bool)
    n136 = Increment(x=w278) -> (x+1=w277:T12)
    n137 = Select(t=w272, s=w273, f=u32 0) -> (s? t:f=w269:u32)
    n138 = case shown="真" w275 {
      tunnel: w279 -> [_ w288]
      tunnel: w277 -> [_ w287]
      frame False {
      }
      frame True {
        n139 = Get Queue Status(queue=w288) -> (queue out=w286:refnum<queue>, # elements in queue=w285:i32)  [unwired: 2 in, 6 out]
        n140 = Equal To 0?(x=w285) -> (x = 0?=w284:bool)
        n141 = case shown="真" w284 {
          tunnel: w287 -> [_ w290]
          tunnel: w286 -> [_ w289]
          frame False {
          }
          frame True {
            n142 = Enqueue Element(queue=w289, element=w290) -> ()  [unwired: 2 in, 3 out]
          }
        }
      }
    }
  }
  n143 = while {
    tunnel: w27 -> [_]
    tunnel: w20 -> [w319]
    stop <- FALSE stop-if-true
    # "时序问题会缺少日志"
    n144 = global read "VARCODMn全局变量.vi" "页面"() -> (w296:enum16{"主页", "参数页", "校准页"})
    n145 = global read "VARCODMn全局变量.vi" "状态告警区"() -> (w347:T8)
    n146 = global read "VARCODMn全局变量.vi" "状态告警区"() -> (w343:T8)
    n147 = global read "VARCODMn全局变量.vi" "状态告警区"() -> (w356:T8)
    n148 = global read "VARCODMn全局变量.vi" "状态告警区"() -> (w322:T8)
    n149 = global read "VARCODMn全局变量.vi" "状态告警区"() -> (w341:T8)
    n150 = global read "VARCODMn全局变量.vi" "时间-温度"() -> (→"时间-温度":u16[])
    n151 = global read "VARCODMn全局变量.vi" "温度曲线"() -> (→"ORP滴定曲线 2":u16[])
    n152 = global read "VARCODMn全局变量.vi" "波形时间"() -> (→"波形时间":timestamp)
    n153 = Wait (ms)(milliseconds to wait=u32 1000 ("等待时间（毫秒）")) -> ()  [unwired: 1 out]
    n154 = case shown="\"校准页\"" w296 {
      tunnel: [_ _ TRUE ("可见")] -> w295
      tunnel: [_ TRUE ("可见") _] -> w294
      frame "主页", Default {
      }
      frame "参数页" {
      }
      frame "校准页" {
      }
    }
    n155 = Unbundle By Name(w356) -> ("id"=w353:u16, "flowid"=w355:u16, "量程"=w354:u16, "工作状态"=w333:u16, "A"=→"A":sgl, "B"=→"B":sgl, "K"=→"K":sgl, "当前滴定数"=→"当前滴定数":sgl, "T"=→"环境温度":sgl, "H"=→"环境湿度":sgl, "运行时间"=→"运行时间":sgl, "当前ORP值"=→"ORP值/光值":sgl, "加热实时温度"=w293:sgl, "当前步骤剩余时间"=→"当前步骤剩余时间":sgl, "结束滴定数"=→"终点滴定数":sgl, "注射泵保温温度"=→"试剂传感器":sgl, "匹配滴定数X0"=→"X0":u16)
    "加热实时温度" <- w293
    n156 = global read "VARCODMn全局变量.vi" "滴定数-ORP值"() -> (→"滴定数-ORP值":u16[])
    n157 = global read "VARCODMn全局变量.vi" "温度波形时间"() -> (→"温度波形时间":timestamp)
    n158 = global read "VARCODMn全局变量.vi" "ORP滴定曲线"() -> (→"ORP滴定曲线":u16[])
    n159 = Unbundle By Name(w343) -> ("工作状态"=w326:u16, "id"=w325:u16)
    n160 = Unbundle By Name(w322) -> ("日志代码"=w338:u16)
    n161 = Unbundle By Name(w341) -> ("日志代码"=w299:u16)
    n162 = Unbundle By Name(w347) -> ("日志代码"=w291:u16, "id"=w346:u16, "故障代码"=w305:u16, "告警代码"=w304:u16)
    n163 = local read "总步数"() -> (w298:i32)
    n164 = case shown="0" w326 {
      frame 0 {
        n165 = local write "数组"(string[] [] ("数组")) -> ()
      }
      frame 1, Default {
      }
    }
    n166 = Divide(x=w299, y=w298) -> (x/y=w301:dbl)
    n167 = feedback #2(w305) -> (w344:u16)
    n168 = feedback-in #2(w305) -> ()
    n169 = feedback #3(w304) -> (w321:u16)
    n170 = feedback-in #3(w304) -> ()
    n171 = feedback-in #4(w338) -> ()
    n172 = feedback #4(w338) -> (w361:u16)
    n173 = feedback #5(w299) -> (w342:u16)
    n174 = feedback-in #5(w299) -> ()
    n175 = Not Equal To 0?(x=w305) -> (x != 0?=w307:bool)
    n176 = Not Equal To 0?(x=w304) -> (x != 0?=w306:bool)
    n177 = Not Equal To 0?(x=w326) -> (x != 0?=w328:bool)
    n178 = Subtract(x=w338, y=1) -> (x-y=→"多列列表框":i32)
    n179 = property on="多列列表框" class="MCListbox (严格)"() -> ("ItemNames"=w317:string[][])  [unwired: 2 in, 2 out]
    n180 = property on="参数查询" class="Bool"("Visible"=w295) -> ()  [unwired: 2 in, 2 out]
    n181 = property on="仪器校准" class="Bool"("Visible"=w294) -> ()  [unwired: 2 in, 2 out]
    n182 = call "消解压力计算.vi"("当前消解温度"=w293) -> ("消解压力"=→"消解压力kPa":dbl)  [unwired: 10 in]
    n183 = Or(x=w307, y=w306) -> (x .or. y?=w303:bool)
    n184 = Not Equal?(x=w344, y=w305) -> (x != y?=w345:bool)
    n185 = Not Equal?(x=w321, y=w304) -> (x != y?=w320:bool)
    n186 = Not Equal?(x=w338, y=w361) -> (x != y?=w360:bool)
    n187 = Not Equal?(x=w299, y=w342) -> (x != y?=w340:bool)
    n188 = call <vilib>:"Boolean Crossing PtByPt.vi"("direction"=enum16{"either", "false-true", "true-false"}."false-true", "input"=w328) -> ("crossing"=w330:bool)  [unwired: 1 in]
    n189 = call <vilib>:"Boolean Crossing PtByPt.vi"("direction"=enum16{"either", "false-true", "true-false"}."true-false", "input"=w328) -> ("crossing"=w327:bool)  [unwired: 1 in]
    n190 = Not Equal To 0?(x=w333) -> (x != 0?=w358:bool)
    n191 = Multiply(x=w301, y=100.0) -> (x*y=→"滑动杆":dbl)
    n192 = case shown="真" w303 {
      tunnel: w346 -> [_ w479]
      tunnel: w345 -> [_ w478]
      tunnel: w320 -> [_ w476]
      tunnel: w304 -> [_ w475]
      tunnel: w319 -> [_ w474]
      tunnel: w305 -> [_ w473]
      tunnel: w291 -> [_ w472]
      frame False {
      }
      frame True {
        n193 = Or(x=w476, y=w478) -> (x .or. y?=w477:bool)
        n194 = case shown="真" w477 {
          tunnel: w479 -> [_ w485]
          tunnel: w473 -> [_ w482]
          tunnel: w475 -> [_ w480]
          tunnel: w474 -> [_ w484]
          tunnel: w472 -> [_ w481]
          frame False {
          }
          frame True {
            n195 = call "id参数转换.vi"("id"=w485) -> ("table输出"=w483:string)  [unwired: 10 in]
            n196 = call "故障告警日志存储 (子VI).vi"("故障代码"=w482, "告警代码"=w480, "日志代码"=w481, "参数"=w483, "队列输入"=w484) -> ()  [unwired: 7 in]
          }
        }
      }
    }
    n197 = case shown="真" w330 {
      tunnel: w325 -> [_ w386]
      tunnel: w326 -> [_ w391]
      frame False {
      }
      frame True {
        n198 = case shown="8" w391 {
          tunnel: [_ "【水样测试】" ("字符串") "【标样核查】" ("字符串") "【零点核查】" ("字符串") "【跨度核查】" ("字符串") "【空白测试】" ("字符串") "【平行样测试】" ("字符串") "【加标回收】" ("字符串") "【空白校准】" ("字符串") "【标样校准】" ("字符串")] -> w390
          frame 0, Default {
          }
          frame 1 {
          }
          frame 2 {
          }
          frame 3 {
          }
          frame 4 {
          }
          frame 5 {
          }
          frame 6 {
          }
          frame 7 {
          }
          frame 8 {
          }
          frame 9 {
          }
        }
        n199 = call "id参数转换.vi"("id"=w386) -> ("table输出"=w385:string)  [unwired: 10 in]
        n200 = Concatenate Strings("<<" ("字符串"), w390, "启动" ("字符串")) -> (w389:string)
        n201 = Get Date/Time In Seconds() -> (seconds since 1Jan1904=w393:timestamp)
        n202 = Bundle By Name(cluster=T14 {"时间标识"=timestamp(0 s since 1904-01-01), "设备"="", "日志信息"="", "流程参数"=""} ("data in"), "时间标识"=w393, "设备"=w385, "日志信息"=w389) -> (w392:T14)
        n203 = call "CODMn操作日志.vi"("data in"=w392) -> ()  [unwired: 11 in]
      }
    }
    n204 = case shown="真" w327 {
      tunnel: w325 -> [_ w368]
      tunnel: w326 -> [_ w372]
      frame False {
      }
      frame True {
        n205 = case shown="1" w372 {
          tunnel: [_ "【水样测试】" ("字符串") "【标样核查】" ("字符串") "【零点核查】" ("字符串") "【跨度核查】" ("字符串") "【空白测试】" ("字符串") "【平行样测试】" ("字符串") "【加标回收】" ("字符串") "【空白校准】" ("字符串") "【标样校准】" ("字符串")] -> w371
          frame 0, Default {
          }
          frame 1 {
          }
          frame 2 {
          }
          frame 3 {
          }
          frame 4 {
          }
          frame 5 {
          }
          frame 6 {
          }
          frame 7 {
          }
          frame 8 {
          }
          frame 9 {
          }
        }
        n206 = call "id参数转换.vi"("id"=w368) -> ("table输出"=w367:string)  [unwired: 10 in]
        n207 = Concatenate Strings(w371, "停止" ("字符串"), ">>" ("字符串")) -> (w370:string)
        n208 = Get Date/Time In Seconds() -> (seconds since 1Jan1904=w374:timestamp)
        n209 = Bundle By Name(cluster=T14 {"时间标识"=timestamp(0 s since 1904-01-01), "设备"="", "日志信息"="", "流程参数"=""} ("data in"), "时间标识"=w374, "设备"=w367, "日志信息"=w370) -> (w373:T14)
        n210 = call "CODMn操作日志.vi"("data in"=w373) -> ()  [unwired: 11 in]
      }
    }
    n211 = Empty Array?(array=w317) -> (empty?=w316:bool)
    n212 = case shown="真" w360 {
      tunnel: w338 -> [_ w507]
      frame False {
      }
      frame True {
        n213 = Subtract(x=w507, y=1) -> (x-y=w505:i32)
        n214 = Subtract(x=w505, y=5) -> (x-y=w509:i32)
        n215 = Greater Or Equal To 0?(x=w509) -> (x >= 0?=w508:bool)
        n216 = property on="多列列表框" class="MCListbox (严格)"() -> (error out=w513:errorcluster, "TopLeft"=w514:T15)  [unwired: 2 in, 1 out]
        n217 = Select(t=w509, s=w508, f=0) -> (s? t:f=w510:i32)
        n218 = Bundle By Name(cluster=w514, "Row"=w510) -> (w515:T15)
        n219 = property on="多列列表框" class="MCListbox (严格)"(error in=w513, "TopLeft"=w515) -> ()  [unwired: 1 in, 2 out]
      }
    }
    n220 = case shown="真" w340 {
      frame False {
      }
      frame True {
        n221 = property on="多列列表框" class="MCListbox (严格)"() -> ("ItemNames"=w408:string[][], "Value"=w409:i32)  [unwired: 2 in, 2 out]
        n222 = Index Array(array=w408, index (row)=w409) -> (element=w407:string[])  [unwired: 1 in]
        n223 = Index Array(array=w407) -> (element=w406:string)  [unwired: 1 in]
        n224 = call "过滤筛选流程.vi"("字符串"=w406) -> ("匹配后偏移量"=w405:i32)  [unwired: 10 in]
        n225 = case shown="默认" w405 {
          tunnel: w406 -> [_ w410]
          frame -1 {
          }
          frame Default {
            # "步骤日志存储"
            n226 = case shown="默认" w410 {
              selector: w410 -> [w416 w418]
              tunnel: [w416 w418] -> w412
              tunnel: [string[] [] ("数组") "数组"] -> w411
              frame "读数" {
              }
              frame Default {
              }
            }
            n227 = for {
              N: 1 -> [_]
              tunnel: w412 -> [w420]
              shift-right: [w419] -> w413
              shift-left: w411 -> [w421]
              n228 = Search 1D Array(1D array=w421, element=w420) -> (index of element=w424:i32)  [unwired: 1 in]
              n229 = Format Into String(format string="%s" ("格式字符串"), w420) -> (resulting string=w425:string)  [unwired: 2 in, 1 out]
              n230 = Equal?(x=w424, y=-1) -> (x = y?=w422:bool)
              n231 = case shown="真" w422 {
                tunnel: w425 -> [_ w433]
                tunnel: w421 -> [w427 w437]
                tunnel: w420 -> [_ w436]
                tunnel: [w427 w435] -> w419
                frame False {
                }
                frame True {
                  n232 = Insert Into Array(array=w437, new element=w436) -> (w435:string[])  [unwired: 1 in]
                  n233 = case shown="\"初始化\"" w433 {
                    selector: w433 -> [w462 w465 w468]
                    tunnel: [w462 w464 w467] -> w429
                    frame Default {
                    }
                    frame "初始化" {
                      n234 = Concatenate Strings("<<" ("字符串"), w465) -> (w464:string)
                    }
                    frame "结束" {
                      n235 = Concatenate Strings(w468, ">>" ("字符串")) -> (w467:string)
                    }
                  }
                  n236 = global read "VARCODMn全局变量.vi" "状态告警区"() -> (w432:T8)
                  n237 = Unbundle By Name(w432) -> ("工作状态"=w431:u16)
                  n238 = case shown="1" w431 {
                    tunnel: [_ "【水样测试】" ("字符串") "【标样核查】" ("字符串") "【零点核查】" ("字符串") "【跨度核查】" ("字符串") "【空白测试】" ("字符串") "【平行样测试】" ("字符串") "【加标回收】" ("字符串") "【空白校准】" ("字符串") "【标样校准】" ("字符串")] -> w430
                    frame 0, Default {
                    }
                    frame 1 {
                    }
                    frame 2 {
                    }
                    frame 3 {
                    }
                    frame 4 {
                    }
                    frame 5 {
                    }
                    frame 6 {
                    }
                    frame 7 {
                    }
                    frame 8 {
                    }
                    frame 9 {
                    }
                  }
                  n239 = global read "VARCODMn全局变量.vi" "状态告警区"() -> (w452:T8)
                  n240 = Unbundle By Name(w452) -> ("id"=w451:u16)
                  n241 = global read "VARCODMn全局变量.vi" "状态告警区"() -> (w447:T8)
                  n242 = case shown="1, 21, 131" w451 {
                    tunnel: [_ "CODMn" ("table输入") "氨氮" ("table输入") "总氮" ("table输入")] -> w449
                    frame Default {
                    }
                    frame 1, 21, 131 {
                    }
                    frame 3, 92 {
                    }
                    frame 2, 76 {
                    }
                  }
                  n243 = Unbundle By Name(w447) -> ("A"=w444:sgl, "B"=w443:sgl, "K"=w442:sgl, "当前滴定数"=w441:sgl, "id"=w440:u16, "flowid"=w439:u16, "量程"=w438:u16)
                  n244 = Concatenate Strings(w430, w429) -> (w428:string)
                  n245 = Format Into String(format string="A=%#f,B=%#f,K=%#f,当前滴定数=%#f,Flow=%d-%-d-%-d" ("格式字符串"), w444, w443, w442, w441, w440, w439, w438) -> (resulting string=w445:string)  [unwired: 2 in, 1 out]
                  n246 = Get Date/Time In Seconds() -> (seconds since 1Jan1904=w448:timestamp)
                  n247 = Bundle By Name(cluster=T14 {"时间标识"=timestamp(0 s since 1904-01-01), "设备"="", "日志信息"="", "流程参数"=""} ("data in"), "时间标识"=w448, "设备"=w449, "日志信息"=w428, "流程参数"=w445) -> (w450:T14)
                  n248 = call "CODMn操作日志.vi"("data in"=w450) -> ()  [unwired: 11 in]
                }
              }
            }
            n249 = local write "数组"(w413) -> ()
          }
        }
      }
    }
    n250 = call <vilib>:"Boolean Crossing PtByPt.vi"("direction"=enum16{"either", "false-true", "true-false"}."either", "input"=w358) -> ("crossing"=w332:bool)  [unwired: 1 in]
    n251 = First Call?() -> (First Call?: T/F=w359:bool)
    n252 = Compound Arithmetic op=OR ("复合运算")(w332, w359, w316) -> (w357:bool)
    n253 = Bundle("id"=w353, "flowid"=w355, "量程"=w354) -> (w348:cluster{"id":u16, "flowid":u16, "量程":u16})  [unwired: 1 in]
    n254 = while {
      tunnel: w357 -> [w493]
      tunnel: w348 -> [w492]
      shift-right: [w489] -> _
      shift-left: _ -> [w490]
      shift-right: [w486] -> _
      shift-left: _ -> [w488]
      stop <- TRUE stop-if-true
      # "XML解析步骤显示"
      n255 = case shown="真" w493 {
        tunnel: [w495 w503] -> w486
        tunnel: [w494 w502] -> w489
        tunnel: w492 -> [_ w497]
        tunnel: w488 -> [w495 _]
        tunnel: w490 -> [w494 _]
        frame False {
        }
        frame True {
          n256 = call "斯坦道XML解析.vi"("添加的路径"="流程路径", "参数簇"=w497) -> ("步骤时间"=w498:string[], "步骤名"=w500:string[])  [unwired: 8 in]
          n257 = for {
            tunnel: w500 -> [_] mode=indexing
            tunnel: [w504] -> w501 mode=indexing
            i -> [w504]
          }
          n258 = Build Array(w500, w498) -> (w499:string[][])
          n259 = Transpose 2D Array(2D array=w499) -> (transposed array=w502:string[][])
          n260 = Number To Decimal String(number=w501) -> (decimal integer string=w503:string[])  [unwired: 1 in]
        }
      }
      n261 = Array Size(array=w486) -> (size(s)=→"总步数":i32)
      n262 = property on="多列列表框" class="MCListbox (严格)"("ItemNames"=w489, "RowHdrs[]"=w486) -> ()  [unwired: 2 in, 2 out]
    }
  }
  n263 = Obtain Queue(name (unnamed)=w6, element data type=cluster{"命令":string, "data":variant} {"命令"="", "data"=variant}) -> (queue out=w18:refnum<queue>)  [unwired: 3 in, 2 out]
  n264 = while {
    tunnel: w18 -> [w522]
    tunnel: [w516] -> _
    stop <- FALSE stop-if-true
    # "定时更新"
    n265 = Get Queue Status(queue=w522) -> (queue out=w520:refnum<queue>, # elements in queue=w519:i32)  [unwired: 2 in, 6 out]
    n266 = call "最小试剂余量百分比.vi"() -> ()  [unwired: 12 in]
    n267 = control-ref of="试剂余量显示"() -> (w517:refnum<vi>)
    n268 = case shown="0" w519 {
      tunnel: w520 -> [_ w526]
      tunnel: [_ w524] -> w516
      frame Default {
      }
      frame 0 {
        n269 = global read "CODMn断电保存全局变量.vi" "站号"() -> (w525:u16)
        n270 = Bundle By Name(cluster=cluster{"命令":string, "data":variant} {"命令"="", "data"=variant} ("元素"), "命令"="读序列号", "data"=w525) -> (w527:cluster{"命令":string, "data":variant})
        n271 = Enqueue Element(queue=w526, element=w527) -> (error out=w524:errorcluster)  [unwired: 2 in, 2 out]
      }
    }
    n272 = Wait (ms)(milliseconds to wait=u32 1000 ("等待时间（毫秒）")) -> ()  [unwired: 1 out]
    n273 = call "试剂余量展示.vi"("波形图 2"=w517) -> ("波形图"=→"试剂余量显示":sgl[][])  [unwired: 10 in]
  }
  n274 = property class="VI"(reference=w17) -> (reference out=w15:refnum<vi>, "Exec.State"=w16:T16)  [unwired: 1 in, 1 out]
  n275 = property class="VI"(reference=w14) -> (reference out=w12:refnum<vi>, "Exec.State"=w13:T16)  [unwired: 1 in, 1 out]
  n276 = case shown="\"Bad\", 默认" w16 {
    tunnel: w15 -> [w530 w534]
    tunnel: [w530 w531] -> w10
    frame "Bad", Default {
    }
    frame "Idle" {
      n277 = invoke class="VI" method="Run VI"(reference=w534, "Wait until done"=FALSE ("结束前等待"), "Auto Dispose Ref"=TRUE ("自动销毁引用")) -> (reference out=w531:refnum<vi>)  [unwired: 2 in, 4 out]
    }
  }
  n278 = case shown="\"Bad\", 默认" w13 {
    tunnel: w12 -> [w535 w539]
    tunnel: [w535 w536] -> w11
    frame "Bad", Default {
    }
    frame "Idle" {
      n279 = invoke class="VI" method="Run VI"(reference=w539, "Wait until done"=FALSE ("结束前等待"), "Auto Dispose Ref"=TRUE ("自动销毁引用")) -> (reference out=w536:refnum<vi>)  [unwired: 2 in, 4 out]
    }
  }
  n280 = call "设置模块队列名.vi"() -> ("Msg"=w7:string)  [unwired: 11 in]
  n281 = Obtain Notifier(name (unnamed)="CODMn" ("名称（未命名）"), notification data type=FALSE) -> (notifier out=w24:refnum<notifier>)  [unwired: 2 in, 2 out]
  n282 = Cancel Notification(0:w24) -> (8:w23:refnum<notifier>)  [unwired: 1 in, 2 out]
  n283 = Obtain Queue(name (unnamed)=w7, element data type=cluster{"命令":string, "data":variant} {"命令"="", "data"=variant}) -> (queue out=w21:refnum<queue>, error out=w32:errorcluster)  [unwired: 3 in, 1 out]
  n284 = while {
    tunnel: w21 -> [w547]
    tunnel: w32 -> [_]
    stop <- FALSE stop-if-true
    n285 = Get Queue Status(queue=w547) -> (queue out=w543:refnum<queue>, # elements in queue=w542:i32)  [unwired: 2 in, 6 out]
    n286 = case shown="0" w542 {
      tunnel: w543 -> [_ w568]
      frame Default {
      }
      frame 0 {
        w556 = u16 0 items=["空闲"=0, "水样测试"=1, "标样核查"=2, "零点核查"=3, "跨度核查"=4, "空白测试"=5, "平行样测试"=6, "加标回收"=7, "空白校准"=8, "标样校准"=9, "初始化（清洗）"=10, "调试"=22, "填充管路"=30, "清洗管路"=31, "清洗反应杯"=32] ("工作状态")
        # "试剂填充 172 \n管路清洗108\n氨氮92\n总磷131\n总磷海水147\n总氮76\n总氮海水92"
        n287 = global read "VARCODMn全局变量.vi" "状态告警区"() -> (w558:T8)
        n288 = global read "CODMn断电保存全局变量.vi" "站号"() -> (w557:u16)
        n289 = Unbundle By Name(w558) -> ("系统时间"=w564:timestamp, "工作状态"=w555:u16)
        n290 = Bundle By Name(cluster=cluster{"命令":string, "data":variant} {"命令"="", "data"=variant} ("元素"), "命令"="读状态告警区", "data"=w557) -> (w566:cluster{"命令":string, "data":variant})
        n291 = Get Date/Time In Seconds() -> (seconds since 1Jan1904=w563:timestamp)
        n292 = Subtract(x=w563, y=w564) -> (x-y=w562:dbl)
        n293 = Equal?(x=w555, y=w556) -> (x = y?=w554:bool)
        n294 = Enqueue Element(queue=w568, element=w566) -> (queue out=w553:refnum<queue>)  [unwired: 2 in, 2 out]
        n295 = case shown="真" w554 {
          tunnel: w557 -> [w570 w578]
          tunnel: w553 -> [w571 w576]
          tunnel: [w569 w575] -> w552
          frame False {
            n296 = Bundle By Name(cluster=cluster{"命令":string, "data":variant} {"命令"="", "data"=variant} ("元素"), "命令"="读滴定曲线", "data"=w570) -> (w572:cluster{"命令":string, "data":variant})
            n297 = Enqueue Element(queue=w571, element=w572) -> (queue out=w569:refnum<queue>)  [unwired: 2 in, 2 out]
          }
          frame True {
            n298 = Bundle By Name(cluster=cluster{"命令":string, "data":variant} {"命令"="", "data"=variant} ("元素"), "命令"="读测量数据区", "data"=w578) -> (w577:cluster{"命令":string, "data":variant})
            n299 = Enqueue Element(queue=w576, element=w577) -> (queue out=w575:refnum<queue>)  [unwired: 2 in, 2 out]
          }
        }
        n300 = Absolute Value(x=w562) -> (abs(x)=w561:dbl)
        n301 = Greater Or Equal?(x=w561, y=30.0) -> (x >= y?=w559:bool)
        n302 = global read "VARCODMn全局变量.vi" "通讯状态"() -> (w550:bool)
        n303 = And(x=w559, y=w550) -> (x .and. y?=w551:bool)
        n304 = case shown="真" w551 {
          tunnel: w552 -> [_ w585]
          tunnel: w557 -> [_ w583]
          frame False {
          }
          frame True {
            n305 = Bundle By Name(cluster=T17 {"站号"=21, "量程切换"=enum."AUTO", "控制命令"=13, "模式设置"=enum."待机", "测量间隔"=0} ("参数"), "站号"=w583) -> (w581:T17)
            n306 = call "CODMn启动命令.vi"("参数"=w581) -> ("启动命令"=w584:cluster{"命令":string, "data":variant})  [unwired: 10 in]
            n307 = Enqueue Element(queue=w585, element=w584) -> ()  [unwired: 2 in, 3 out]
          }
        }
      }
    }
    n308 = Wait (ms)(milliseconds to wait=u32 1000 ("等待时间（毫秒）")) -> ()  [unwired: 1 out]
    n309 = global read "CODMn断电保存全局变量.vi" "流程路径"() -> (w546:path)
    n310 = local write "流程路径"(w546) -> ()
    n311 = global read "CODMn断电保存全局变量.vi" "MB通信方式选择"() -> (w544:enum16{"串口", "TCP"})
    n312 = global read "CODMn断电保存全局变量.vi" "远程标样校准"() -> (w541:enum16{"标液1", "标液2", "标液3", "标液4"})
    n313 = global read "CODMn断电保存全局变量.vi" "远程校准量程"() -> (w540:enum16{"低量程1", "低量程2", "高量程1", "高量程2"})
    n314 = local write "平台反控标样校准"(w541) -> ()
    n315 = local write "平台反控校准量程"(w540) -> ()
    n316 = case shown="\"TCP\"" w544 {
      tunnel: [w586 w587] -> w545
      frame "串口", Default {
        n317 = global read "CODMn断电保存全局变量.vi" "VISA Resource"() -> (w586:refnum<visa-resource-name>)
      }
      frame "TCP" {
        n318 = global read "CODMn断电保存全局变量.vi" "IP"() -> (w587:string)
      }
    }
    "字符串" <- w545
  }
  n319 = control-ref of="测量模式下拉列表"() -> (w29:refnum<vi>)
  n320 = control-ref of="参数下拉列表"() -> (w30:refnum<vi>)
  n321 = control-ref of="量程下拉列表"() -> (w31:refnum<vi>)
  n322 = control-ref of="公式"() -> (w28:refnum<vi>)
  n323 = while {
    tunnel: w21 -> [w596]
    tunnel: w31 -> [w595]
    tunnel: w30 -> [w594]
    tunnel: w29 -> [w593]
    tunnel: w28 -> [w592]
    tunnel: w23 -> [w591]
    tunnel: [w590] -> _
    tunnel: w11 -> [w589]
    tunnel: w10 -> [w588]
    stop <- FALSE stop-if-true
    n324 = event shown="[9] \"手动启动\": 值改变" {
      selector: _ -> [_ _ _ _ _ _ _ _ _ _ _ _ _ _ _ _ _ _ _ _ _ _]
      dyn-events: _ -> [_ _ _ _ _ _ _ _ _ _ _ _ _ _ _ _ _ _ _ _ _ _]
      timeout: _ -> [_ _ _ _ _ _ _ _ _ _ _ _ _ _ _ _ _ _ _ _ _ _]
      tunnel: w596 -> [_ _ _ _ _ _ _ _ _ w648 _ w666 _ _ _ _ _ _ _ _ _ _]
      tunnel: w595 -> [_ _ _ _ w610 _ _ w627 _ _ _ _ _ _ _ _ _ _ _ _ _ _]
      tunnel: w594 -> [_ _ _ _ w609 _ _ w623 _ _ _ _ _ _ _ _ _ _ _ _ w739 w745]
      tunnel: w593 -> [_ _ _ _ w608 _ _ w625 _ _ _ _ _ _ _ _ _ _ _ _ _ _]
      tunnel: w592 -> [_ _ _ _ w611 _ _ w621 _ _ _ _ _ _ _ _ _ _ _ _ _ _]
      tunnel: w591 -> [_ _ _ _ _ _ _ _ _ _ _ w669 _ _ _ _ _ _ _ _ _ _]
      tunnel: [_ _ _ _ w606 _ _ _ _ _ _ _ _ _ _ _ _ _ _ _ _ _] -> w590
      tunnel: w589 -> [_ _ _ _ _ _ _ _ _ _ _ _ w672 _ _ _ _ _ _ _ _ _]
      tunnel: w588 -> [_ _ _ _ _ _ _ _ _ _ _ _ _ w676 _ _ _ _ _ _ _ _]
      event Timeout {
        n325 = event-data() -> ()  [unwired: 1 in, 3 out]
      }
      event "布尔": Value Change {
        n326 = event-data() -> ("NewVal"=w598:bool)  [unwired: 1 in, 5 out]
        n327 = case shown="假" w598 {
          frame False {
            n328 = global write "VARCODMn全局变量.vi" "权限等级"(enum16{"一级权限", "二级权限", "三级权限", "超级权限"}."一级权限" ("权限等级")) -> ()
          }
          frame True {
            n329 = global read "VARCODMn全局变量.vi" "权限密码"() -> (w602:u32[])
            n330 = global read "VARCODMn全局变量.vi" "权限等级"() -> (w601:enum16{"一级权限", "二级权限", "三级权限", "超级权限"})
            n331 = call "密码权限设置.vi"("权限输入"=w601, "权限密码"=w602) -> ("权限输出"=w600:enum16{"一级权限", "二级权限", "三级权限", "超级权限"})  [unwired: 9 in]
            n332 = global write "VARCODMn全局变量.vi" "权限等级"(w600) -> ()
          }
        }
      }
      event "权限等级": Mouse Down {
        n333 = event-data() -> ()  [unwired: 1 in, 8 out]
        n334 = global read "VARCODMn全局变量.vi" "权限密码"() -> (w605:u32[])
        n335 = global read "VARCODMn全局变量.vi" "权限等级"() -> (w604:enum16{"一级权限", "二级权限", "三级权限", "超级权限"})
        n336 = call "密码权限设置.vi"("权限输入"=w604, "权限密码"=w605) -> ("权限输出"=w603:enum16{"一级权限", "二级权限", "三级权限", "超级权限"})  [unwired: 9 in]
        n337 = global write "VARCODMn全局变量.vi" "权限等级"(w603) -> ()
      }
      event "流程固件": Value Change {
        n338 = event-data() -> ()  [unwired: 1 in, 6 out]
        n339 = call "流程固件设置对话框.vi"() -> ()  [unwired: 12 in]
      }
      event "测量模式下拉列表", "量程下拉列表", "参数下拉列表": Value Change {
        n340 = event-data() -> ()  [unwired: 1 in, 6 out]
        n341 = property class="Enum (严格)"(reference=w609) -> ("Value"=w615:enum16{"CODMn"})  [unwired: 1 in, 2 out]
        n342 = property class="Enum (严格)"(reference=w610) -> ("Value"=w614:enum16{"低量程1", "低量程2", "高量程1", "高量程2"})  [unwired: 1 in, 2 out]
        n343 = property class="Enum (严格)"(reference=w608) -> ("Value"=w612:T3)  [unwired: 1 in, 2 out]
        n344 = call "公式读取.vi"("量程"=w614, "测量模式"=w612, "测量参数"=w615) -> ("error out"=w606:errorcluster, "临界滴定数"=w607:dbl, "公式"=w613:cluster{"X^2":dbl, "X":dbl, "b":dbl})  [unwired: 6 in]
        n345 = property class="Clust (严格)"(reference=w611, "Value"=w613) -> ()  [unwired: 1 in, 2 out]
        n346 = local write "公式切换阈值滴定数(0~9999)"(w607) -> ()
      }
      event "平台反控校准量程", "平台反控标样校准": Value Change {
        n347 = event-data() -> ()  [unwired: 1 in, 6 out]
        n348 = flat-sequence {
          frame #0 {
            n349 = global write "CODMn断电保存全局变量.vi" "远程标样校准"("平台反控标样校准") -> ()
            n350 = global write "CODMn断电保存全局变量.vi" "远程校准量程"("平台反控校准量程") -> ()
          }
          frame #1 {
            n351 = call "配置文件保存.vi"() -> ()  [unwired: 12 in]
          }
        }
      }
      event "流程路径": Value Change {
        n352 = event-data() -> ()  [unwired: 1 in, 6 out]
        n353 = flat-sequence {
          frame #0 {
            n354 = local read "流程路径"() -> (w618:path)
            n355 = global write "CODMn断电保存全局变量.vi" "流程路径"(w618) -> ()
          }
          frame #1 {
            n356 = call "配置文件保存.vi"() -> ()  [unwired: 12 in]
          }
        }
      }
      event "公式单个写入": Value Change {
        n357 = event-data() -> ()  [unwired: 1 in, 6 out]
        n358 = property class="Enum (严格)"(reference=w623) -> ("Value"=w622:enum16{"CODMn"})  [unwired: 1 in, 2 out]
        n359 = property class="Enum (严格)"(reference=w627) -> ("Value"=w626:enum16{"低量程1", "低量程2", "高量程1", "高量程2"})  [unwired: 1 in, 2 out]
        n360 = property class="Enum (严格)"(reference=w625) -> ("Value"=w624:T3)  [unwired: 1 in, 2 out]
        n361 = property class="Clust (严格)"(reference=w621) -> ("Value"=w620:cluster{"X^2":dbl, "X":dbl, "b":dbl})  [unwired: 1 in, 2 out]
        n362 = call "公式写入.vi"("公式"=w620, "量程"=w626, "测量模式"=w624, "测量参数"=w622) -> ("error out"=w628:errorcluster)  [unwired: 7 in]
        n363 = case shown="无错误" w628 {
          tunnel: w624 -> [w637 _]
          tunnel: w626 -> [w635 _]
          tunnel: w620 -> [w631 _]
          tunnel: ["写入成功" ("消息") "写入失败" ("消息")] -> w619
          frame No Error {
            n364 = Equal?(x=w637, y=T3."水样测量") -> (x = y?=w634:bool)
            n365 = Equal?(x=w635, y=enum16{"低量程", "高量程"}."低量程" ("量程下拉列表")) -> (x = y?=w633:bool)
            n366 = And(x=w634, y=w633) -> (x .and. y?=w632:bool)
            n367 = case shown="真" w632 {
              tunnel: w631 -> [_ w638]
              frame False {
              }
              frame True {
                n368 = Unbundle By Name(w638) -> ("X^2"=w641:dbl, "X"=w640:dbl, "b"=w639:dbl)
                n369 = global read "CODMn断电保存全局变量.vi" "CODMn仪器参数"() -> (w642:T18)
                n370 = Bundle By Name(cluster=w642, "曲线截距"=w639, "曲线斜率"=w640, "二次多项式系数"=w641) -> (w643:T18)
                n371 = global write "CODMn断电保存全局变量.vi" "CODMn仪器参数"(w643) -> ()
              }
            }
          }
          frame Error {
          }
        }
        n372 = One Button Dialog(message=w619) -> ()  [unwired: 1 in, 1 out]
      }
      event "试剂余量设置": Value Change {
        n373 = event-data() -> ()  [unwired: 1 in, 6 out]
        n374 = call "试剂余量显示UI.vi"() -> ()  [unwired: 12 in]
      }
      event "手动启动": Value Change {
        n375 = event-data() -> ()  [unwired: 1 in, 6 out]
        n376 = call "CODMn启动参数对话框.vi"() -> ("标样浓度输出"=w646:dbl, "确认"=w645:bool, "元素"=w647:cluster{"命令":string, "data":variant})  [unwired: 9 in]
        n377 = case shown="真" w645 {
          tunnel: w648 -> [_ w658]
          tunnel: w647 -> [_ w657]
          tunnel: w646 -> [_ w650]
          frame False {
          }
          frame True {
            (unwired) u16 31 ("y")
            n378 = Enqueue Element(queue=w658, element=w657) -> ()  [unwired: 2 in, 3 out]
            n379 = global write "VARCODMn全局变量.vi" "手动启动"(TRUE ("手动启动")) -> ()
            n380 = Unbundle By Name(w657) -> ("data"=w656:variant)
            n381 = Variant To Data(type=cluster{"站号":u16, "控制命令":u16[]} {"站号"=0, "控制命令"=[]} ("输出簇"), Variant=w656) -> (data=w654:cluster{"站号":u16, "控制命令":u16[]})  [unwired: 1 in, 1 out]
            n382 = Unbundle By Name(w654) -> ("控制命令"=w653:u16[])
            n383 = Index Array(array=w653) -> (element=w652:u16)  [unwired: 1 in]
            n384 = Swap Bytes(anything=w652) -> (byte swapped=w651:u16)
            n385 = case shown="31" w651 {
              tunnel: w650 -> [_ w659 _ _ _]
              frame 0, Default {
              }
              frame 2 {
                # "标样核查"
                n386 = flat-sequence {
                  tunnel: w659 -> [w660]
                  frame #0 {
                    n387 = global read "CODMn断电保存全局变量.vi" "质控参数设置"() -> (w662:T19)
                    n388 = Bundle By Name(cluster=w662, "标准液标准浓度"=w660) -> (w661:T19)
                    n389 = global write "CODMn断电保存全局变量.vi" "质控参数设置"(w661) -> ()
                  }
                  frame #1 {
                    n390 = call "配置文件保存.vi"() -> ()  [unwired: 12 in]
                  }
                }
              }
              frame 8 {
                # "空白校准"
                n391 = property on="量程下拉列表" class="Enum (严格)"("Val(Sgnl)"=enum16{"低量程1", "低量程2", "高量程1", "高量程2"}."低量程1" ("值(信号)")) -> ()  [unwired: 2 in, 2 out]
              }
              frame 9 {
                # "标样校准"
                n392 = local read "平台反控校准量程"() -> (w664:enum16{"低量程1", "低量程2", "高量程1", "高量程2"})
                n393 = property on="量程下拉列表" class="Enum (严格)"("Val(Sgnl)"=w664) -> ()  [unwired: 2 in, 2 out]
              }
              frame 31 {
                n394 = One Button Dialog(message="“请将纯水管置于纯水中，其余管路置于清洗废液桶中”" ("消息")) -> ()  [unwired: 1 in, 1 out]
              }
            }
          }
        }
      }
      event "单步测试": Value Change {
        n395 = event-data() -> ()  [unwired: 1 in, 6 out]
        n396 = call "COMn单步调试对话框.vi"() -> ()  [unwired: 12 in]
      }
      event "停止": Value Change {
        n397 = event-data() -> ()  [unwired: 1 in, 6 out]
        n398 = Enqueue Element(queue=w666, element=cluster{"命令":string, "data":variant} {"命令"="启动", "data"=variant(cluster{"站号":u16, "控制命令":u16[]} {"站号"=21, "控制命令"=[2816]})} ("启动命令")) -> ()  [unwired: 2 in, 3 out]
        n399 = Cancel Notification(0:w669) -> (8:w670:refnum<notifier>)  [unwired: 1 in, 2 out]
        n400 = Send Notification(notification=TRUE ("通知"), notifier=w670) -> ()  [unwired: 1 in, 2 out]
      }
      event "设置", "参数查询": Value Change {
        n401 = event-data() -> ()  [unwired: 1 in, 6 out]
        n402 = invoke on="子面板" class="SubPnl" method="Remove VI"() -> (error out=w673:errorcluster)  [unwired: 3 in, 2 out]
        n403 = property on="窗格" class="Pane"("Origin"=T6 {"Horizontal"=0, "Vertical"=628} ("原点")) -> ()  [unwired: 2 in, 2 out]
        n404 = global write "VARCODMn全局变量.vi" "页面"(enum16{"主页", "参数页", "校准页"}."参数页" ("页面")) -> ()
        n405 = invoke on="子面板" class="SubPnl" method="Insert VI"(error in=w673, "VI Ref"=w672) -> ()  [unwired: 2 in, 4 out]
      }
      event "仪器校准": Value Change {
        n406 = event-data() -> ()  [unwired: 1 in, 6 out]
        n407 = invoke on="子面板" class="SubPnl" method="Remove VI"() -> (error out=w677:errorcluster)  [unwired: 3 in, 2 out]
        n408 = global write "VARCODMn全局变量.vi" "页面"(enum16{"主页", "参数页", "校准页"}."校准页" ("页面")) -> ()
        n409 = invoke on="子面板" class="SubPnl" method="Insert VI"(error in=w677, "VI Ref"=w676) -> ()  [unwired: 2 in, 4 out]
      }
      event "滴定曲线": Value Change {
        n410 = event-data() -> ()  [unwired: 1 in, 6 out]
        n411 = vi-ref "读取CODMn数据波形新.vi"() -> (w679:refnum<vi>)
        n412 = property class="VI"(reference=w679) -> ("Name"=w685:string)  [unwired: 1 in, 2 out]
        n413 = Open VI Reference(type specifier VI Refnum (for type only)=refnum<vi> refnum, vi path=w685, options=128 ("选项")) -> (vi reference=w683:refnum<vi>, error out=w682:errorcluster)  [unwired: 3 in]
        n414 = call-by-ref "?"(reference=w683, error in=w682) -> (reference out=w680:refnum<vi>, error out=w681:errorcluster)  [unwired: 12 in]
        n415 = Close Reference(reference=w680, error in (no error)=w681) -> ()  [unwired: 1 out]
      }
      event "历史波形", "历史波形 2": Value Change {
        n416 = event-data() -> ("CtlRef"=w687:refnum<vi>)  [unwired: 1 in, 5 out]
        n417 = property class="Bool (严格)"(reference=w687) -> ("Label.Text"=w686:string)  [unwired: 1 in, 2 out]
        n418 = call-poly <vilib>:"Read Waveforms from File.vi"() -> ("error out"=w688:errorcluster, "first waveform in record"=w689:waveform(dbl))  [unwired: 6 in, 2 out]
        n419 = case shown="无错误" w688 {
          tunnel: w689 -> [w693 _]
          tunnel: w686 -> [w690 _]
          frame No Error {
            n420 = Unbundle By Name(w693) -> ("t0"=w692:timestamp, "Y"=w691:dbl[])  [unwired: 2 out]
            n421 = case shown="\"历史波形\", 默认" w690 {
              tunnel: w692 -> [w694 w697]
              tunnel: w691 -> [w695 w696]
              frame "历史波形2" {
                n422 = global write "VARCODMn全局变量.vi" "温度波形时间"(w694) -> ()
                n423 = global write "VARCODMn全局变量.vi" "温度曲线"(w695) -> ()
                n424 = global write "VARCODMn全局变量.vi" "时间-温度"(w695) -> ()
              }
              frame "历史波形", Default {
                n425 = global write "VARCODMn全局变量.vi" "波形时间"(w697) -> ()
                n426 = global write "VARCODMn全局变量.vi" "ORP滴定曲线"(w696) -> ()
                n427 = global write "VARCODMn全局变量.vi" "滴定数-ORP值"(w696) -> ()
              }
            }
          }
          frame Error {
            n428 = One Button Dialog(message="打开失败" ("消息")) -> ()  [unwired: 1 in, 1 out]
          }
        }
      }
      event "返回", "返回 2", "返回 3": Value Change {
        n429 = event-data() -> ()  [unwired: 1 in, 6 out]
        n430 = global write "VARCODMn全局变量.vi" "页面"(enum16{"主页", "参数页", "校准页"}."主页" ("页面")) -> ()
        n431 = property on="窗格" class="Pane"("Origin"=T6 {"Horizontal"=0, "Vertical"=0} ("原点")) -> ()  [unwired: 2 in, 2 out]
      }
      event "公式.X^2", "公式.X", "公式.b", "公式切换阈值滴定数(0~9999)": Mouse Down {
        n432 = event-data() -> ("CtlRef"=w704:refnum<vi>)  [unwired: 1 in, 5 out]
        n433 = property class="DigNum (严格)"(reference=w704) -> (reference out=w702:refnum<vi>, "Value"=w703:dbl)  [unwired: 1 in, 1 out]
        n434 = call "数字键盘.vi"("OldNumber"=w703) -> ("NewNumber"=w701:dbl)
        n435 = property class="DigNum (严格)"(reference=w702, "Val(Sgnl)"=w701) -> ()  [unwired: 1 in, 2 out]
      }
      event "读公式": Value Change {
        n436 = event-data() -> ()  [unwired: 1 in, 6 out]
      }
      event "写公式": Value Change {
        n437 = event-data() -> ()  [unwired: 1 in, 6 out]
        n438 = Two Button Dialog(message="即将将左侧拟合公式写入仪器所有模式\n请选择是否写入?" ("消息"), 1:"否" ("F按钮名称（“取消”）"), 2:"是" ("T按钮名称（“确定”）")) -> (T button?=w705:bool)
        n439 = case shown="真" w705 {
          frame False {
          }
          frame True {
            n440 = for {
              N: 7 -> [_]
              shift-right: [w714] -> _
              shift-left: T3."水样测量" ("测量模式下拉列表") -> [w715]
              tunnel: [w713] -> w709
              n441 = call "公式写入.vi"("临界滴定数"="公式切换阈值滴定数(0~9999)", "公式"="公式", "量程"="量程下拉列表", "测量模式"=w715, "测量参数"="参数下拉列表") -> ("error out"=w719:errorcluster)  [unwired: 6 in]
              n442 = Increment(x=w715) -> (x+1=w714:T3)
              n443 = case shown="无错误" w719 {
                tunnel: w715 -> [w728 _]
                tunnel: "量程下拉列表" -> [w727 _]
                tunnel: "公式" -> [w723 _]
                tunnel: ["写入成功" ("消息") "写入失败" ("消息")] -> w713
                frame No Error {
                  n444 = Equal?(x=w728, y=T3."水样测量") -> (x = y?=w726:bool)
                  n445 = Equal?(x=w727, y=enum16{"低量程1", "低量程2", "高量程1", "高量程2"}."低量程1") -> (x = y?=w725:bool)
                  n446 = And(x=w726, y=w725) -> (x .and. y?=w724:bool)
                  n447 = case shown="真" w724 {
                    tunnel: w723 -> [_ w729]
                    frame False {
                    }
                    frame True {
                      n448 = Unbundle By Name(w729) -> ("X^2"=w732:dbl, "X"=w731:dbl, "b"=w730:dbl)
                      n449 = global read "CODMn断电保存全局变量.vi" "CODMn仪器参数"() -> (w733:T18)
                      n450 = Bundle By Name(cluster=w733, "曲线截距"=w730, "曲线斜率"=w731, "二次多项式系数"=w732) -> (w734:T18)
                      n451 = global write "CODMn断电保存全局变量.vi" "CODMn仪器参数"(w734) -> ()
                    }
                  }
                }
                frame Error {
                }
              }
            }
            n452 = One Button Dialog(message=w709) -> ()  [unwired: 1 in, 1 out]
          }
        }
      }
      event "量程切换阈值读取": Value Change {
        n453 = event-data() -> ()  [unwired: 1 in, 6 out]
        n454 = property class="Enum (严格)"(reference=w739) -> ("Value"=w738:enum16{"CODMn"})  [unwired: 1 in, 2 out]
        n455 = call "量程读取.vi"("测量参数"=w738) -> ("error out"=w736:errorcluster)  [unwired: 9 in, 1 out]
        n456 = case shown="错误" w736 {
          tunnel: ["读取成功" ("消息") "读取失败" ("消息")] -> w737
          frame No Error {
          }
          frame Error {
          }
        }
        n457 = One Button Dialog(message=w737) -> ()  [unwired: 1 in, 1 out]
      }
      event "量程切换阈值写入": Value Change {
        n458 = event-data() -> ()  [unwired: 1 in, 6 out]
        n459 = property class="Enum (严格)"(reference=w745) -> ("Value"=w744:enum16{"CODMn"})  [unwired: 1 in, 2 out]
        n460 = call "量程写入.vi"("测量参数"=w744) -> ("error out"=w742:errorcluster)  [unwired: 9 in]
        n461 = case shown="无错误" w742 {
          tunnel: ["写入成功" ("消息") "写入失败" ("消息")] -> w743
          frame No Error {
          }
          frame Error {
          }
        }
        n462 = One Button Dialog(message=w743) -> ()  [unwired: 1 in, 1 out]
      }
    }
  }
  n463 = call "Close TimingControl.vi"("error in (no error)"=w1, "TimingControl in"=w2) -> ()  [unwired: 9 in, 1 out]
